vi "CUST Get PMU Real Data.vi"(7 "Channel Info":T1, 10 "pseudoPdcId":i32, 11 "pmuIndex":i32) -> (0 "function return":i32, 1 "Digital Values":bool[](array[boolean]), 2 "Analog Values":sgl[](array[numeric]), 3 "Phasor Values":csg[](array[numeric]), 4 "Frequency":sgl, 5 "status":T2, 6 "Delta Frequency":sgl)   [LabVIEW 2013, in "C37118-DLL.lvlib"]
doc: "STRONGRIDIEEEC37118DLL_API int __cdecl getPmuRealDataLabview(noArraysPmuDataFrame* rd, PmuStatus* status,\n uint16_t PhasorArrayLength, float* phasorValueReal, float* phasorValueImaginary,\n uint16_t AnalogArrayLength, float* analogValueArr,\n uint16_t DigitalArrayLength, uint8_t* digitalValueArr,\n int32_t pseudoPdcId, int32_t pmuIndex);\n\nSTRONGRIDIEEEC37118DLL_API int __cdecl getPmuRealDataLabview(noArraysPmuDataFrame* rd, PmuStatus* status,\n uint16_t PhasorArrayLength, float* phasorValueReal, float* phasorValueImaginary,\n uint16_t AnalogArrayLength, float* analogValueArr,\n uint16_t DigitalArrayLength, uint8_t* digitalValueArr,\n int32_t pseudoPdcId, int32_t pmuIndex);"
uses:
  C37118-DLL.lvlib
  builds/StrongridDLL/StrongridDLL.dll
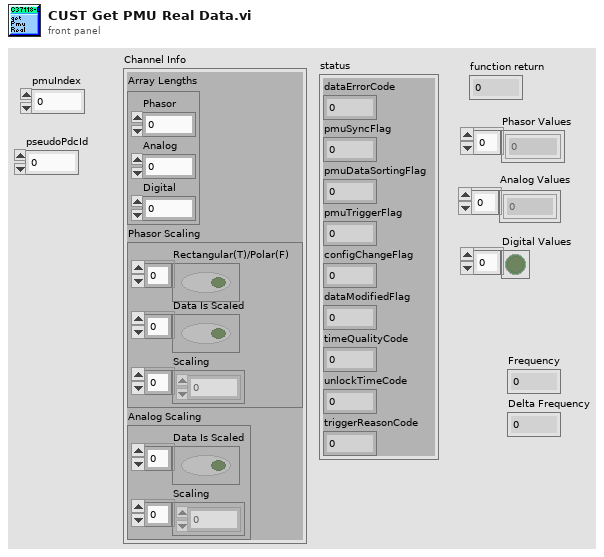
[diagram p1: front panel]
types:
  T1 = cluster{"Array Lengths":cluster{"Phasor":i32, "Analog":i32, "Digital":i32}, "Phasor Scaling":cluster{"Rectangular(T)/Polar(F)":bool[], "Data Is Scaled":bool[], "Scaling":sgl[]}, "Analog Scaling":cluster{"Data Is Scaled":bool[], "Scaling":sgl[]}}
  T2 = cluster{"dataErrorCode":u8, "pmuSyncFlag":u8, "pmuDataSortingFlag":u8, "pmuTriggerFlag":u8, "configChangeFlag":u8, "dataModifiedFlag":u8, "timeQualityCode":u8, "unlockTimeCode":u8, "triggerReasonCode":u8}
  T3 = cluster{"Phasor":i32, "Analog":i32, "Digital":i32}
  T4 = cluster{"Rectangular(T)/Polar(F)":bool[], "Data Is Scaled":bool[], "Scaling":sgl[]}
  T5 = cluster{"Data Is Scaled":bool[], "Scaling":sgl[]}
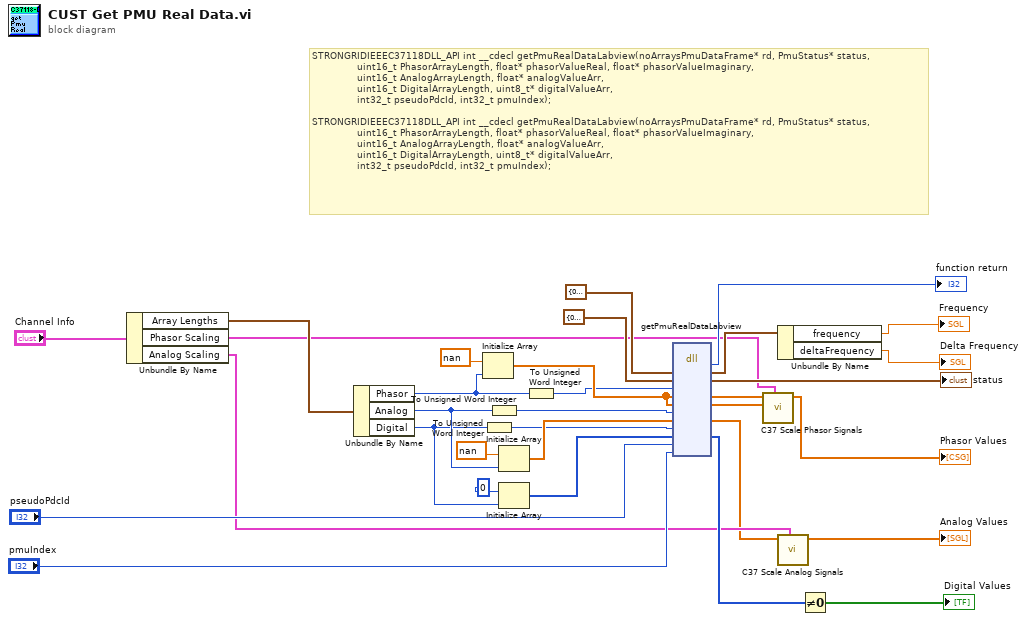
[diagram p0: block diagram]
diagram:
  # "STRONGRIDIEEEC37118DLL_API int __cdecl getPmuRealDataLabview(noArraysPmuDataFrame* rd, PmuStatus* status,\n               uint16_t PhasorArrayLength, float* phasorValueReal, float* phasorValueImaginary,\n               uint16_t AnalogArrayLength, float* analogValueArr,\n               uint16_t DigitalArrayLength, uint8_t* digitalValueArr,\n               int32_t pseudoPdcId, int32_t pmuIndex);\n\nSTRONGRIDIEEEC37118DLL_API int __cdecl getPmuRealDataLabview(noArraysPmuDataFrame* rd, PmuStatus* status,\n\t\t\t\t\t\t\t\t\t\t\t\t\t\t\tuint16_t PhasorArrayLength, float* phasorValueReal, float* phasorValueImaginary,\n\t\t\t\t\t\t\t\t\t\t\t\t\t\t\tuint16_t AnalogArrayLength, float* analogValueArr,\n\t\t\t\t\t\t\t\t\t\t\t\t\t\t\tuint16_t DigitalArrayLength, uint8_t* digitalValueArr,\n\t\t\t\t\t\t\t\t\t\t\t\t\t\t\tint32_t pseudoPdcId, int32_t pmuIndex);"
  n1 = Unbundle By Name("Channel Info") -> ("Array Lengths"=w9:T3, "Phasor Scaling"=w4:T4, "Analog Scaling"=w3:T5)
  n2 = Unbundle By Name(w9) -> ("Phasor"=w21:i32, "Analog"=w17:i32, "Digital"=w14:i32)
  n3 = Initialize Array(sgl nan ("frequency"), w21) -> (w19:sgl[])
  n4 = To Unsigned Word Integer(number=w14) -> (unsigned 16bit integer=w10:u16)
  n5 = To Unsigned Word Integer(number=w17) -> (unsigned 16bit integer=w11:u16)
  n6 = Initialize Array(sgl nan ("frequency"), w17) -> (w16:sgl[])
  n7 = Initialize Array(i8 0 ("frequency"), w14) -> (w13:i8[])
  n8 = To Unsigned Word Integer(number=w21) -> (unsigned 16bit integer=w12:u16)
  n9 = dll-call lib="C:/dev/OSS/S3DK/builds/StrongridDLL/StrongridDLL.*" fn="getPmuRealDataLabview"("rd"=cluster{"frequency":sgl, "deltaFrequency":sgl} {"frequency"=0.0, "deltaFrequency"=0.0}, "status"=T2 {"dataErrorCode"=0, "pmuSyncFlag"=0, "pmuDataSortingFlag"=0, "pmuTriggerFlag"=0, "configChangeFlag"=0, "dataModifiedFlag"=0, "timeQualityCode"=0, "unlockTimeCode"=0, "triggerReasonCode"=0}, "PhasorArrayLength"=w12, "phasorValueReal"=w19, "phasorValueImaginary"=w19, "AnalogArrayLength"=w11, "analogValueArr"=w16, "DigitalArrayLength"=w10, "digitalValueArr"=w13, "pseudoPdcId"="pseudoPdcId", "pmuIndex"="pmuIndex") -> ("return type"=→"function return":i32, "rd"=w29:cluster{"frequency":sgl, "deltaFrequency":sgl}, "status"=→"status":T2, "phasorValueReal"=w7:sgl[], "phasorValueImaginary"=w6:sgl[], "analogValueArr"=w2:sgl[], "digitalValueArr"=w25:i8[])  [unwired: 8 in, 2 out]
  n10 = call "C37 Scale Phasor Signals.vi"("Phasor Scaling"=w4, "Phasor Value Imaginary (or angle)"=w6, "Phasor Value Real (or amplitude)"=w7) -> ("Phasor Values"=→"Phasor Values":csg[])  [unwired: 7 in, 1 out]
  n11 = Unbundle By Name(w29) -> ("frequency"=→"Frequency":sgl, "deltaFrequency"=→"Delta Frequency":sgl)
  n12 = call "C37 Scale Analog Signals.vi"("Analog Scaling"=w3, "Analog Values"=w2) -> ("Scaled Analog Values"=→"Analog Values":sgl[])  [unwired: 9 in]
  n13 = Not Equal To 0?(x=w25) -> (x != 0?=→"Digital Values":bool[])
